vi "StreamEngine.ExitCmd.Send.vi"(8 "error in (no error)":errorcluster, 11 "Q Refs":T1) -> (0 "error out":errorcluster)   [LabVIEW 2025, in "XNET Bus Monitor Client.lvlib"]
uses:
  XNET Bus Monitor Client.lvlib
  Types/StreamEngine.CmdQueueData.Cmd.ctl
  Types/StreamEngine.CmdQueueData.ctl
  Types/StreamEngine.QueueRefs.ctl
  Types/SubProcessEngine.CmdQueueData.ctl
  Types/SubProcessEngine.CmdQueueData.Cmd.ctl
  Types/SubProcessEngine.QueueRefs.ctl
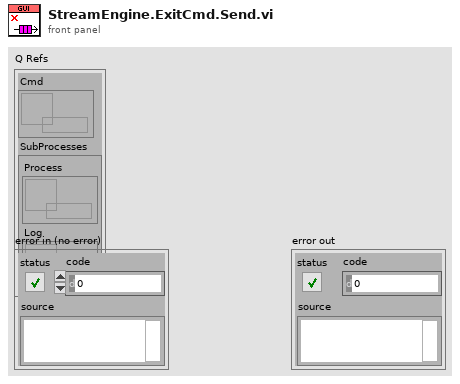
[diagram p1: front panel]
types:
  T1 = typedef "XNET Bus Monitor Client.lvlib/StreamEngine.QueueRefs.ctl" = cluster{"Cmd":refnum<queue>, "SubProcesses":T2}
  T2 = typedef "XNET Bus Monitor Client.lvlib/SubProcessEngine.QueueRefs.ctl" = cluster{"Process":refnum<queue>, "Log":refnum<queue>}
  T3 = typedef "XNET Bus Monitor Client.lvlib/StreamEngine.CmdQueueData.ctl" = cluster{"Cmd":T4, "Parameters":variant}
  T4 = typedef "XNET Bus Monitor Client.lvlib/StreamEngine.CmdQueueData.Cmd.ctl" = enum8{"Start Stream", "Stop Stream", "Exit"}
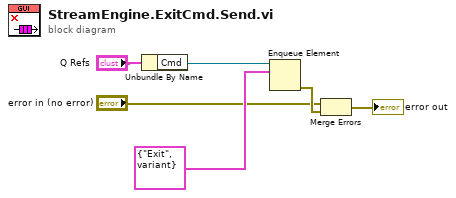
[diagram p0: block diagram]
diagram:
  n1 = Unbundle By Name("Q Refs") -> ("Cmd"=w1:refnum<queue>)
  n2 = Enqueue Element(queue=w1, element=T3 {"Cmd"=enum."Exit", "Parameters"=variant(path path "")}) -> (error out=w4:errorcluster)  [unwired: 2 in, 2 out]
  n3 = Merge Errors("error in (no error)", w4) -> (→"error out":errorcluster)
